vi "prompt_file_saving.vi"(1 "safe time steps":bool, 2 "safe combined spectra":bool, 3 "safe spectra steps":bool, 7 "start exp":bool) -> (8 "Start Experiment":bool)   [LabVIEW 2012]
doc: "This vi's displays a warning if no measurement data will be saved."
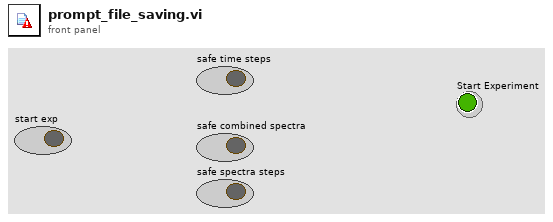
[diagram p1: front panel]
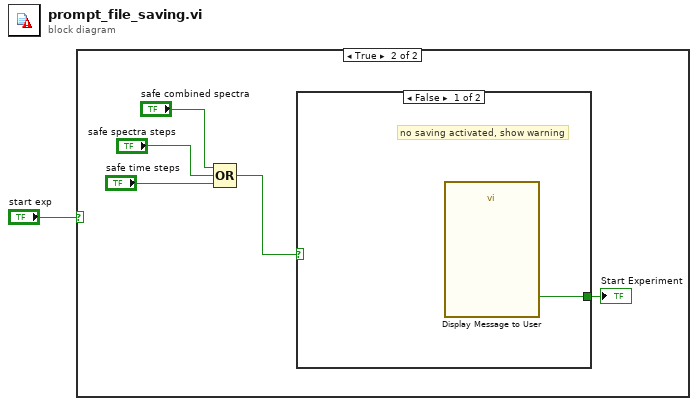
[diagram p0: block diagram]
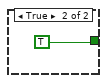
[diagram p3: hidden frame]
diagram:
  n1 = case shown="True" "start exp" {
    frame False {
    }
    frame True {
      n2 = Compound Arithmetic op=OR("safe combined spectra", "safe spectra steps", "safe time steps") -> (w3:bool)
      n3 = case shown="False" w3 {
        tunnel: [w7 TRUE] -> w2
        frame False {
          # "no saving activated, show warning"
          n4 = call "Display Message to User"() -> ("Start Experiment"=w7:bool)  [unwired: 10 in, 1 out]
        }
        frame True {
        }
      }
      "Start Experiment" <- w2
    }
  }
